vi "DAQ-AI Mean Value.vi"(8 "Cluster":T1, 11 "data":dbl[][](array[numeric]) format="%0.2f") -> (3 "Analoge Input":dbl[](array[numeric]))   [LabVIEW 2015]
uses:
  <vilib>/Analysis/baseanly.llb/Mean (DBL).vi
  Galobal variable_TI.vi
  <vilib>/Analysis/NI_AALBase.lvlib
  <vilib>/ptbypt/NI_PtbyPt.lvlib
panel:
  out "AI_as DI":bool[](array[boolean])
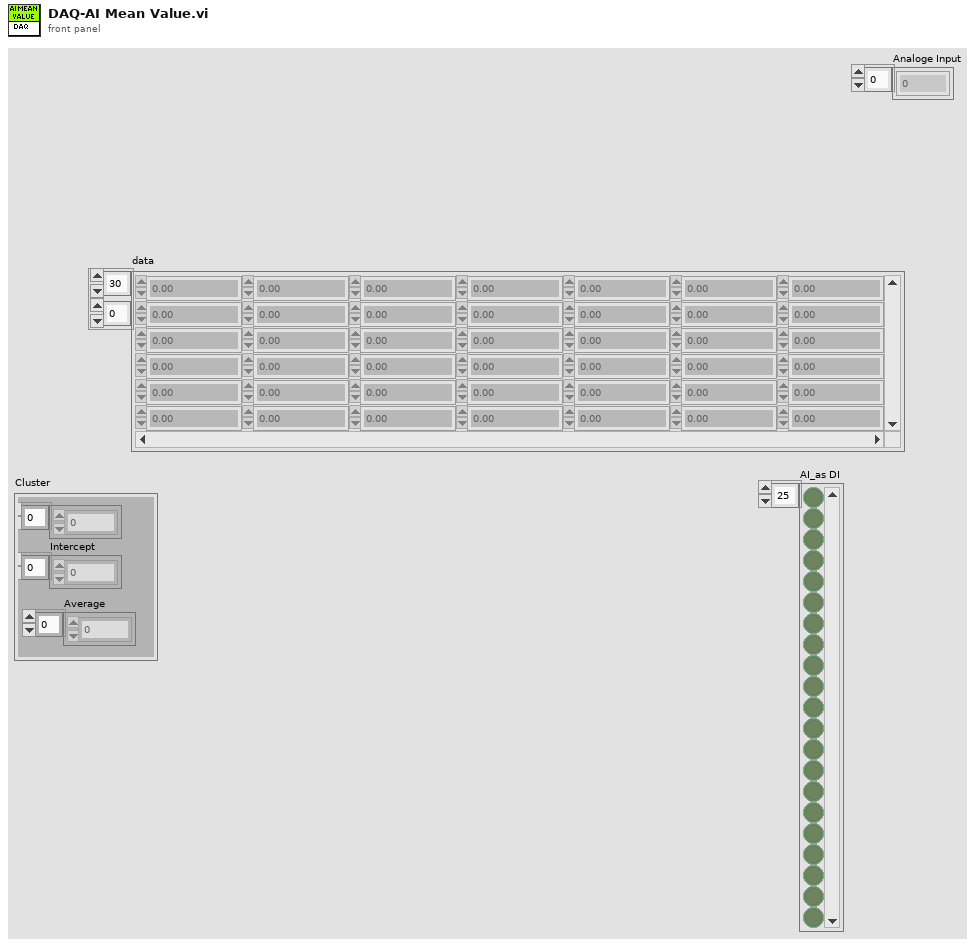
[diagram p1: front panel]
types:
  T1 = cluster{"Slop":dbl[], "Intercept":dbl[], "Average ":i16[]}
  T2 = typedef "Control 11.ctl" = dbl
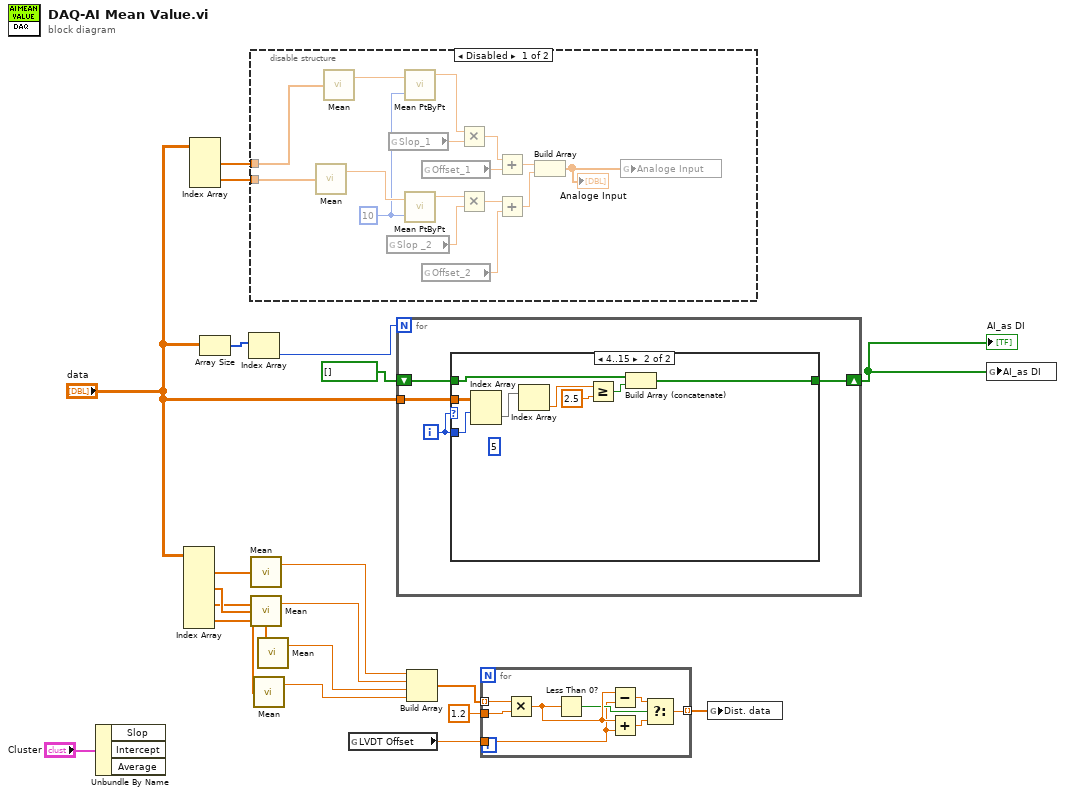
[diagram p0: block diagram]
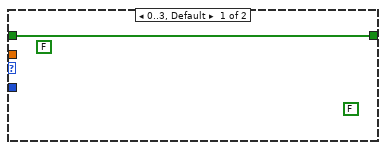
[diagram p3: hidden frame]
diagram:
  n1 = Unbundle By Name("Cluster") -> ()  [unwired: 3 out]
  n2 = Index Array(array="data") -> (element #1=w13:dbl[], element #2=w12:dbl[], element #3=w10:dbl[], element #4=w9:dbl[])  [unwired: 8 in]
  n3 = Index Array(array="data") -> (element #1=w17:dbl[], element #2=w20:dbl[])  [unwired: 4 in]
  n4 = Array Size(array="data") -> (size(s)=w19:i32[])
  n5 = Index Array(array=w19) -> (element=w16:i32)  [unwired: 1 in]
  n6 = disable-structure shown="Disabled" {
    disable-tunnel: w20 -> [w36 _]
    disable-tunnel: w17 -> [w33 _]
    frame Disabled {
      w32 = 10 ("sample length")
      n7 = call-poly <vilib>:"Mean.vi"("X"=w36) -> ("mean"=w34:dbl)  [unwired: 1 out]
      n8 = call-poly <vilib>:"Mean.vi"("X"=w33) -> ("mean"=w35:dbl)  [unwired: 1 out]
      n9 = global read "Galobal variable_TI.vi" "Slop _2"() -> (w24:dbl)
      n10 = global read "Galobal variable_TI.vi" "Slop_1"() -> (w29:dbl)
      n11 = call <vilib>:"Mean PtByPt.vi"("x"=w35, "sample length"=w32) -> ("mean"=w30:dbl)  [unwired: 2 in, 1 out]
      n12 = call <vilib>:"Mean PtByPt.vi"("x"=w34, "sample length"=w32) -> ("mean"=w25:dbl)  [unwired: 2 in, 1 out]
      n13 = global read "Galobal variable_TI.vi" "Offset_1"() -> (w27:dbl)
      n14 = global read "Galobal variable_TI.vi" "Offset_2"() -> (w23:dbl)
      n15 = Multiply(x=w30, y=w29) -> (x*y=w28:dbl)
      n16 = Multiply(x=w25, y=w24) -> (x*y=w26:dbl)
      n17 = Add(x=w28, y=w27) -> (x+y=w22:dbl)
      n18 = Add(x=w26, y=w23) -> (x+y=w21:dbl)
      n19 = Build Array(w22, w21) -> (w31:dbl[])
      "Analoge Input" <- w31
      n20 = global write "Galobal variable_TI.vi" "Analoge Input"(w31) -> ()
    }
    frame Enabled {
    }
  }
  n21 = call-poly <vilib>:"Mean.vi"("X"=w13) -> ("mean"=w5:dbl)  [unwired: 1 out]
  n22 = call-poly <vilib>:"Mean.vi"("X"=w12) -> ("mean"=w4:dbl)  [unwired: 1 out]
  n23 = call-poly <vilib>:"Mean.vi"("X"=w9) -> ("mean"=w2:dbl)  [unwired: 1 out]
  n24 = call-poly <vilib>:"Mean.vi"("X"=w10) -> ("mean"=w3:dbl)  [unwired: 1 out]
  n25 = global read "Galobal variable_TI.vi" "LVDT Offset"() -> (w1:T2)
  n26 = for {
    N: w16 -> [_]
    tunnel: "data" -> [w40]
    shift-right: [w38] -> w15
    shift-left: bool[] [] -> [w37]
    i -> [w39]
    n27 = case shown="4..15" w39 {
      tunnel: w40 -> [_ w49]
      tunnel: w39 -> [_ w45]
      tunnel: [w41 w43] -> w38
      tunnel: w37 -> [w41 w42]
      frame 0..3, Default {
        (unwired) FALSE
        (unwired) FALSE
      }
      frame 4..15 {
        (unwired) 5
        n28 = Index Array(array=w49, index (row)=w45) -> (element=w46:dbl[])  [unwired: 1 in]
        n29 = Index Array(array=w46) -> (element=w48:dbl)  [unwired: 1 in]
        n30 = Greater Or Equal?(x=w48, y=2.5) -> (x >= y?=w44:bool)
        n31 = Build Array (concatenate)(w42, w44) -> (w43:bool[])
      }
    }
  }
  "AI_as DI" <- w15
  n32 = Build Array(w5, w4, w3, w2) -> (w8:dbl[])
  n33 = for {
    tunnel: w8 -> [w56] mode=indexing
    tunnel: [w51] -> w7 mode=indexing
    tunnel: 1.2 ("y") -> [w57]
    tunnel: w1 -> [w50]
    n34 = Multiply(x=w56, y=w57) -> (x*y=w55:dbl)
    n35 = Less Than 0?(x=w55) -> (x < 0?=w54:bool)
    n36 = Subtract(x=w55, y=w50) -> (x-y=w53:T2)
    n37 = Add(x=w55, y=w50) -> (x+y=w52:T2)
    n38 = Select(t=w53, s=w54, f=w52) -> (s? t:f=w51:T2)
  }
  n39 = global write "Galobal variable_TI.vi" "Dist. data"(w7) -> ()
  n40 = global write "Galobal variable_TI.vi" "AI_as DI"(w15) -> ()
